vi "tacking_math.vi"() -> (3 "Sailling Pts":cluster{"X":dbl, "Y":dbl}[](array[cluster]))   [LabVIEW 2013]
doc: "Calculates the nextoptimal tacking location, given:\n the waypoint and wind in the boat's frame of reference\n the maximum distance to travel before tacking\n the current estimated number of tacks needed to reach the waypoint\n and irons range\n\n(11/5/2014) Kaitlin Gallagher and Rocco Diverdi"
uses:
  <vilib>/Analysis/baseanly.llb/Real A x B.vi
  <vilib>/Analysis/NI_AALBase.lvlib
panel:
  in  "number of tacks":dbl
  out "Y":dbl
  out "X":dbl
  in  "Max Tack Length":dbl
  in  "Irons Range":dbl
  in  "Wind":dbl
  in  "Waypoint":cluster{"X":dbl, "Y":dbl}
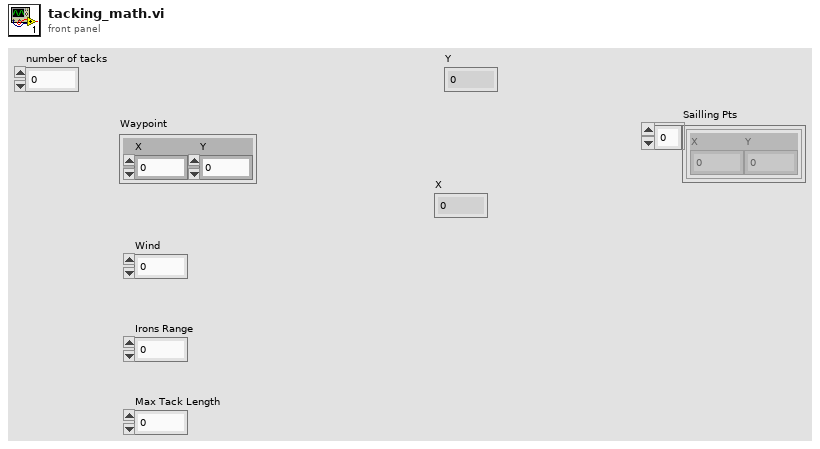
[diagram p1: front panel]
types:
  T1 = typedef "NI_Matrix.lvlib/RealMatrix.ctl" = dbl[][]
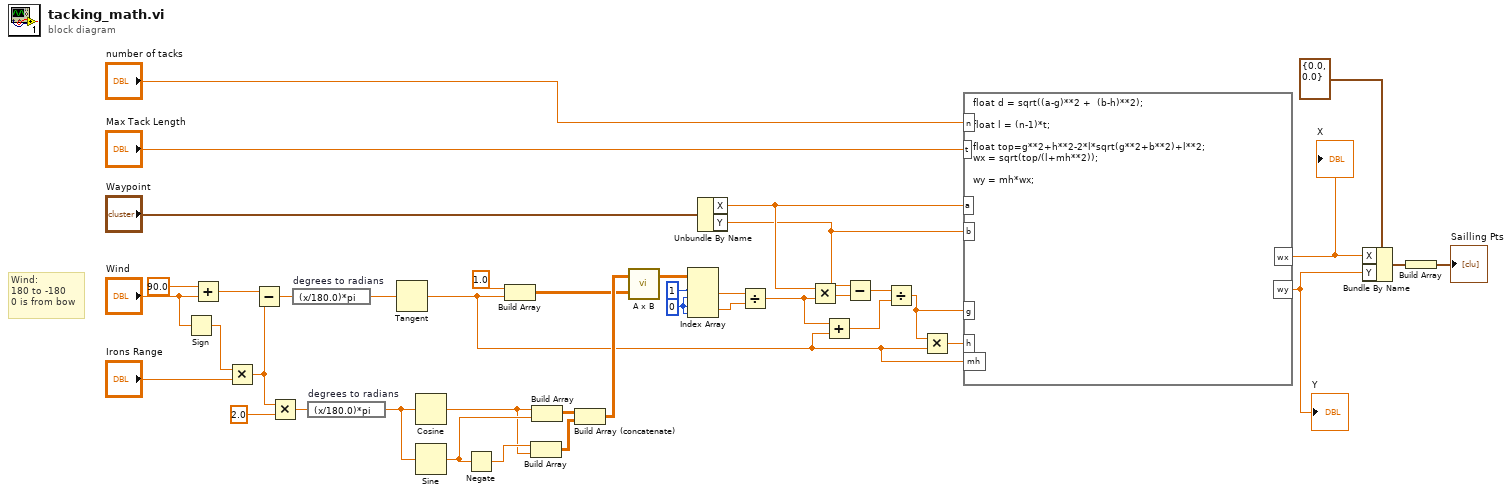
[diagram p0: block diagram]
diagram:
  w18 = 0 ("index (row)")
  # "Wind:\n180 to -180\n0 is from bow"
  n1 = Sign(1:"Wind") -> (0:w38:dbl)
  n2 = Add(x=90.0, y="Wind") -> (x+y=w39:dbl)
  n3 = Multiply(x=w38, y="Irons Range") -> (x*y=w2:dbl)
  n4 = Subtract(x=w39, y=w2) -> (x-y=w36:dbl)
  n5 = Multiply(x=w2, y=2.0 ("x")) -> (x*y=w25:dbl)
  n6 = expression code="(x/180.0)*pi" "degrees to radians"(w36) -> (w35:dbl)
  n7 = expression code="(x/180.0)*pi" "degrees to radians"(w25) -> (w24:dbl)
  n8 = Tangent(1:w35) -> (0:w9:dbl)
  n9 = Cosine(x=w24) -> (cos(x)=w30:dbl)
  n10 = Sine(x=w24) -> (sin(x)=w32:dbl)
  n11 = Negate(x=w32) -> (-x=w31:dbl)
  n12 = Build Array(1.0, w9) -> (w26:T1)
  n13 = Build Array(w31, w30) -> (w28:T1)
  n14 = Build Array(w30, w32) -> (w29:T1)
  n15 = Build Array (concatenate)(w29, w28) -> (w27:T1)
  n16 = call-poly <vilib>:"A x B.vi"("B"=w26, "A"=w27) -> ("A x B"=w23:T1)  [unwired: 1 out]
  n17 = Index Array(array=w23, index (row) #1=1 ("index (row)"), index (col) #1=w18, index (row) #2=w18, index (col) #2=w18) -> (element #1=w21:dbl, element #2=w20:dbl)
  n18 = Unbundle By Name("Waypoint") -> ("X"=w12:dbl, "Y"=w11:dbl)
  n19 = Divide(x=w21, y=w20) -> (x/y=w17:dbl)
  n20 = Multiply(x=w12, y=w17) -> (x*y=w19:dbl)
  n21 = Add(x=w17, y=w9) -> (x+y=w15:dbl)
  n22 = Subtract(x=w11, y=w19) -> (x-y=w16:dbl)
  n23 = Divide(x=w16, y=w15) -> (x/y=w13:dbl)
  n24 = Multiply(x=w13, y=w9) -> (x*y=w14:dbl)
  n25 = formula code="float d = sqrt((a-g)**2 +  (b-h)**2);\n\nfloat l = (n-1)*t;\n\nfloat top=g**2+h**2-2*l*sqrt(g**2+b**2)+l**2;\nwx = sqrt(top/(l+mh**2));\n\nwy = mh*wx;"("a"=w12, "b"=w11, "g"=w13, "h"=w14, "t"="Max Tack Length", "mh"=w9, "n"="number of tacks") -> ("wx"=w7:dbl, "wy"=w5:dbl)
  "X" <- w7
  "Y" <- w5
  n26 = Bundle By Name(cluster=cluster{"Y":dbl, "X":dbl} {"Y"=0.0, "X"=0.0} ("Waypoint"), "X"=w7, "Y"=w5) -> (w4:cluster{"Y":dbl, "X":dbl})
  n27 = Build Array(w4) -> (→"Sailling Pts":cluster{"Y":dbl, "X":dbl}[])
